vi "Get Chassis Info.vi"(8 "error in":errorcluster, 11 "Session in":refnum<k21>="localhost") -> (0 "error out":errorcluster, 2 "Chassis Information":T1[](array[typedef]) {"Modules"."Module Code" format="%.0x"; "Product ID" format="%.0x"}, 3 "Session out":refnum<k21>="localhost")   [LabVIEW 2016]
uses:
  <resource>/objmgr/niflexriosae.rc
  <resource>/objmgr/nicriosae.rc
  <vilib>/nisyscfg/nisyscfg.lvlib
  <vilib>/nisyscfg/Close (Hardware).vi
  <vilib>/nisyscfg/Close (Filter).vi
  Chassis/Controls/ChassisInformation.ctl
  Chassis/Chassis.lvclass
  Controls/ChassisInformation.ctl
  RT Management.lvclass
  Module/Controls/ModuleInformation.ctl
  Module/Module.lvclass
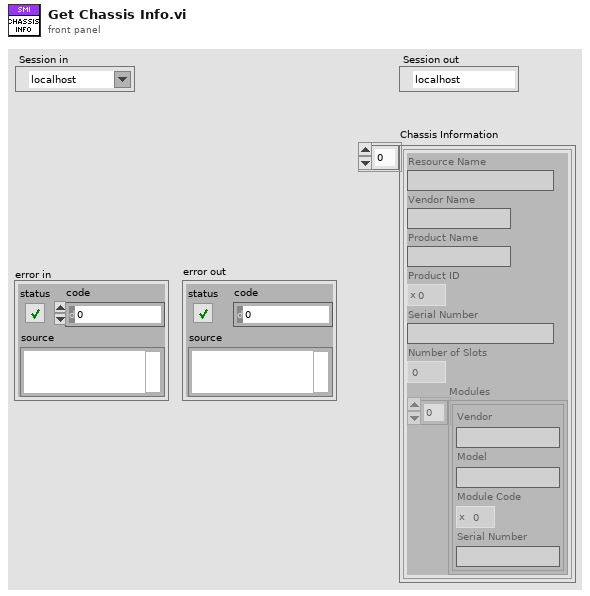
[diagram p1: front panel]
types:
  T1 = typedef "RT Management.lvlib/RT Management.lvclass/ChassisInformation.ctl" = cluster{"Resource Name":string, "Vendor Name":string, "Product Name":string, "Product ID":u32, "Serial Number":string, "Number of Slots":i32, "Modules":T2[]}
  T2 = typedef "SMI.lvlib/Module.lvclass/ModuleInformation.ctl" = cluster{"Vendor":string, "Model":string, "Module Code":u16, "Serial Number":string}
  T3 = typedef "SMI.lvlib/Chassis.lvclass/ChassisInformation.ctl" = cluster{"Resource Name":string, "Vendor Name":string, "Product Name":string, "Product ID":u16, "Serial Number":string, "Number of Slots":i32}
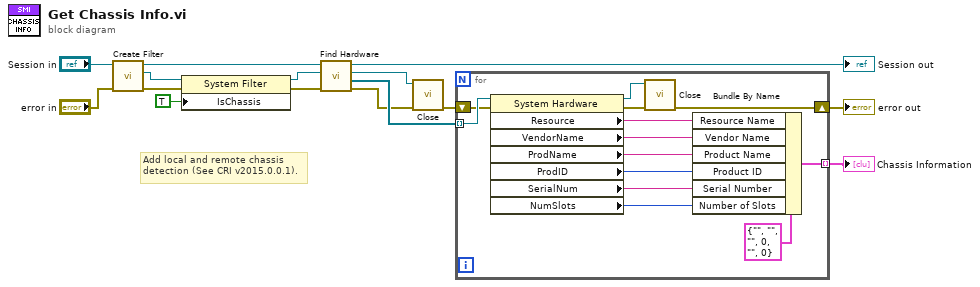
[diagram p0: block diagram]
diagram:
  # "Add local and remote chassis\ndetection (See CRI v2015.0.0.1)."
  n1 = call <vilib>:"Create Filter.vi"("error in (no error)"="error in", "Session in"="Session in") -> ("error out"=w9:errorcluster, "Filter out"=w10:refnum<k20>, "Session out"=w11:refnum<k21>)  [unwired: 7 in]
  n2 = property class="System Filter"(reference=w10, error in=w9, "IsChassis"=TRUE ("Is Chassis")) -> (reference out=w12:refnum<k20>, error out=w13:errorcluster)
  n3 = call <vilib>:"Find Hardware.vi"("error in (no error)"=w13, "Filter in"=w12, "Session in"=w11) -> ("error out"=w5:errorcluster, "Resources out"=w6:refnum<k20>[], "Filter out"=w15:refnum<k20>, "Session out"=→"Session out":refnum<k21>)  [unwired: 5 in]
  n4 = call-poly <vilib>:"Close.vi"("error in (no error)"=w5, "Filter in"=w15) -> ("error out"=w4:errorcluster)  [unwired: 9 in]
  n5 = for {
    tunnel: w6 -> [w27] mode=indexing
    shift-right: [w25] -> w2
    shift-left: w4 -> [w26]
    tunnel: [w28] -> w3 mode=indexing
    n6 = property class="System Hardware"(reference=w27, error in=w26) -> (reference out=w24:refnum<k20>, error out=w17:errorcluster, "Resource"=w22:string, "VendorName"=w21:string, "ProdName"=w20:string, "ProdID"=w19:u32, "SerialNum"=w18:string, "NumSlots"=w16:i32)
    n7 = call-poly <vilib>:"Close.vi"("error in (no error)"=w17, "Resource in"=w24) -> ("error out"=w25:errorcluster)  [unwired: 9 in]
    n8 = Bundle By Name(cluster=T3 {"Resource Name"="", "Vendor Name"="", "Product Name"="", "Product ID"=0, "Serial Number"="", "Number of Slots"=0} ("Chassis Information"), "Resource Name"=w22, "Vendor Name"=w21, "Product Name"=w20, "Product ID"=w19, "Serial Number"=w18, "Number of Slots"=w16) -> (w28:T3)
  }
  "error out" <- w2
  "Chassis Information" <- w3
